vi "mac_mem_dot_32bit_mem_row1_12_outside.vi"(0 "StartIndex":u8, 1 "x_i":T2, 2 "Boolean":bool) -> (16 "ziyi_type":T1)   [LabVIEW 2017]
uses:
  x_qp_scalar.ctl
  ziyi_pipe.ctl
  typeDefs/QP_mem_type.ctl
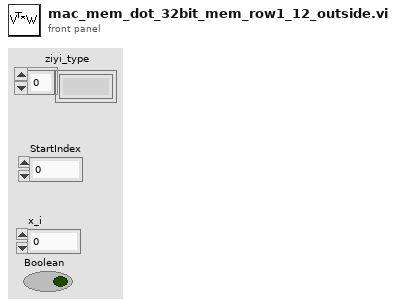
[diagram p1: front panel]
types:
  T1 = typedef "ziyi_pipe.ctl" = T2[]
  T2 = typedef "x_qp_scalar.ctl" = fxp<+/-,32,6>
  T3 = typedef "QP_mem_type.ctl" = refnum<k21>
  T4 = typedef "xtype_scalar.ctl" = fxp<+/-,32,6>
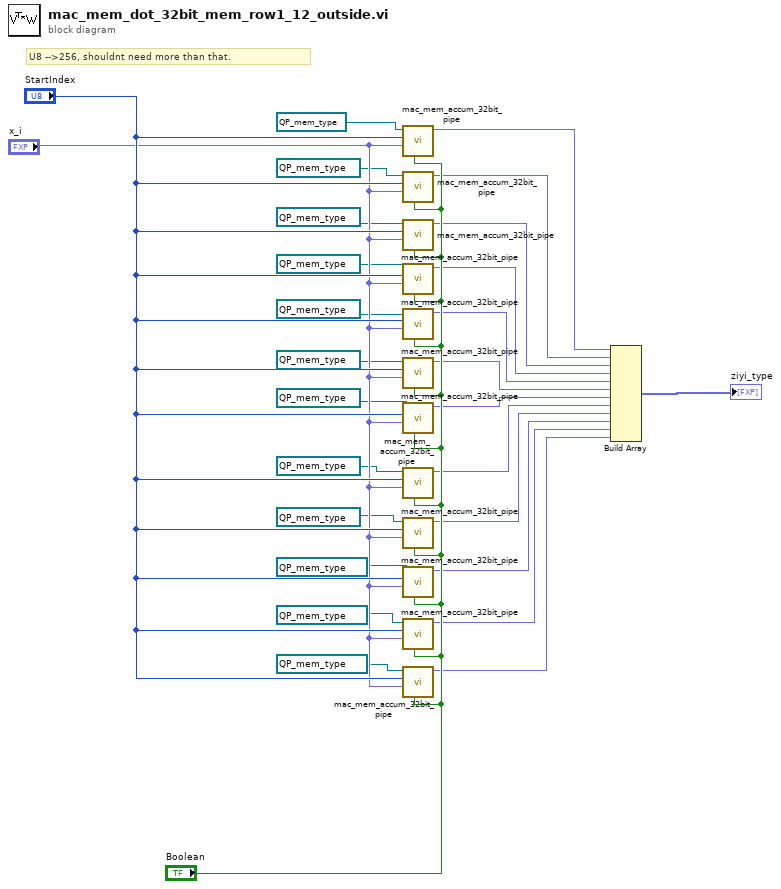
[diagram p0: block diagram]
diagram:
  # "U8 -->256, shouldnt need more than that."
  n1 = call "mac_mem_accum_32bit_pipe.vi"("sclr"="Boolean", "x_i"="x_i", "readIndex"="StartIndex", "QP-Memory"=T3 "Memory" ("Memory In")) -> ("s"=w25:T4)  [unwired: 7 in]
  n2 = call "mac_mem_accum_32bit_pipe.vi"("sclr"="Boolean", "x_i"="x_i", "readIndex"="StartIndex", "QP-Memory"=T3 "Memory 2" ("Memory In")) -> ("s"=w24:T4)  [unwired: 7 in]
  n3 = call "mac_mem_accum_32bit_pipe.vi"("sclr"="Boolean", "x_i"="x_i", "readIndex"="StartIndex", "QP-Memory"=T3 "Memory 3" ("Memory In")) -> ("s"=w23:T4)  [unwired: 7 in]
  n4 = call "mac_mem_accum_32bit_pipe.vi"("sclr"="Boolean", "x_i"="x_i", "readIndex"="StartIndex", "QP-Memory"=T3 "Memory 4" ("Memory In")) -> ("s"=w22:T4)  [unwired: 7 in]
  n5 = call "mac_mem_accum_32bit_pipe.vi"("sclr"="Boolean", "x_i"="x_i", "readIndex"="StartIndex", "QP-Memory"=T3 "Memory 5" ("Memory In")) -> ("s"=w21:T4)  [unwired: 7 in]
  n6 = call "mac_mem_accum_32bit_pipe.vi"("sclr"="Boolean", "x_i"="x_i", "readIndex"="StartIndex", "QP-Memory"=T3 "Memory 6" ("Memory In")) -> ("s"=w20:T4)  [unwired: 7 in]
  n7 = call "mac_mem_accum_32bit_pipe.vi"("sclr"="Boolean", "x_i"="x_i", "readIndex"="StartIndex", "QP-Memory"=T3 "Memory 7" ("Memory In")) -> ("s"=w19:T4)  [unwired: 7 in]
  n8 = call "mac_mem_accum_32bit_pipe.vi"("sclr"="Boolean", "x_i"="x_i", "readIndex"="StartIndex", "QP-Memory"=T3 "Memory 8" ("Memory In")) -> ("s"=w18:T4)  [unwired: 7 in]
  n9 = call "mac_mem_accum_32bit_pipe.vi"("sclr"="Boolean", "x_i"="x_i", "readIndex"="StartIndex", "QP-Memory"=T3 "Memory 9" ("Memory In")) -> ("s"=w17:T4)  [unwired: 7 in]
  n10 = call "mac_mem_accum_32bit_pipe.vi"("sclr"="Boolean", "x_i"="x_i", "readIndex"="StartIndex", "QP-Memory"=T3 "Memory 10" ("Memory In")) -> ("s"=w16:T4)  [unwired: 7 in]
  n11 = call "mac_mem_accum_32bit_pipe.vi"("sclr"="Boolean", "x_i"="x_i", "readIndex"="StartIndex", "QP-Memory"=T3 "Memory 11" ("Memory In")) -> ("s"=w15:T4)  [unwired: 7 in]
  n12 = call "mac_mem_accum_32bit_pipe.vi"("sclr"="Boolean", "x_i"="x_i", "readIndex"="StartIndex", "QP-Memory"=T3 "Memory 12" ("Memory In")) -> ("s"=w14:T4)  [unwired: 7 in]
  n13 = Build Array(w25, w24, w23, w22, w21, w20, w19, w18, w17, w16, w15, w14) -> (→"ziyi_type":T4[])
